vi "Attack.vi"(8 "error in (no error)":errorcluster, 9 "Attack?":T1, 10 "Team Index":i32, 11 "View":i32[](array[numeric])) -> (0 "error out":errorcluster, 1 "Direction":i32, 2 "Action":T2, 3 "View":i32[](array[numeric]), 4 "Enemy Found?":bool, 6 "Enemy Direction":i32)   [LabVIEW 2015, in "Common.lvlib"]
uses:
  Common.lvlib
  Type Defs/Action Enum.ctl
  Formics/Attack Options.ctl
  Type Defs/SB Type Defs.lvlib
  Formics/Formics.lvclass
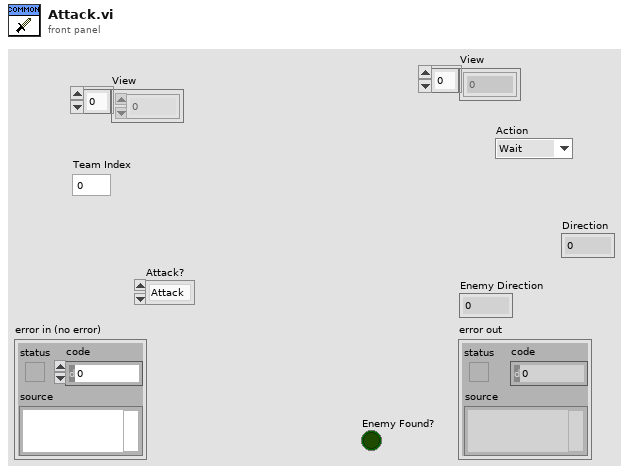
[diagram p1: front panel]
types:
  T1 = typedef "Formics.lvclass/Attack Options.ctl" = enum16{"Attack", "Run", "Distract"}
  T2 = typedef "SB Type Defs.lvlib/Action Enum.ctl" = enum16{"Wait", "Move", "Attack", "Replicate"}
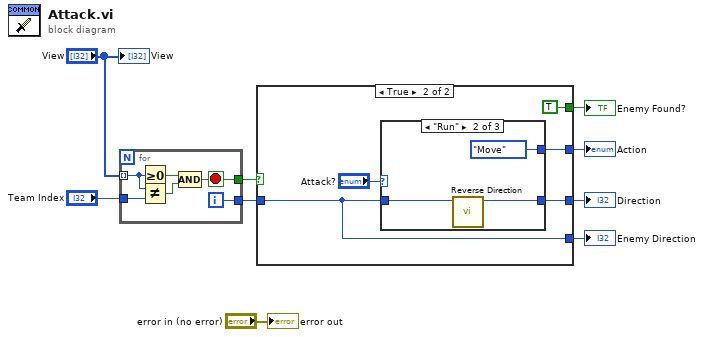
[diagram p0: block diagram]
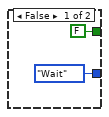
[diagram p2: hidden frame]
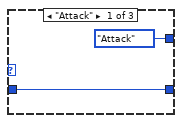
[diagram p3: hidden frame]
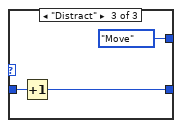
[diagram p4: hidden frame]
diagram:
  n1 = for {
    tunnel: "View" -> [w13] mode=indexing
    tunnel: "Team Index" -> [w14]
    tunnel: [w11] -> w2
    tunnel: [w10] -> w1
    i -> [w11]
    stop <- w10 stop-if-true
    n2 = Greater Or Equal To 0?(x=w13) -> (x >= 0?=w15:bool)
    n3 = Not Equal?(x=w13, y=w14) -> (x != y?=w12:bool)
    n4 = Compound Arithmetic op=AND(w15, w12) -> (w10:bool)
  }
  n5 = case shown="True" w1 {
    tunnel: [Action_Enum."Wait" ("Action") w22] -> w7
    tunnel: [_ w20] -> w8
    tunnel: [FALSE ("Enemy Found?") TRUE ("Enemy Found?")] -> w6
    tunnel: [_ w18] -> w5
    tunnel: w2 -> [_ w18]
    frame False {
    }
    frame True {
      n6 = case shown="\"Run\"" "Attack?" {
        tunnel: [Action_Enum."Attack" ("Action") Action_Enum."Move" ("Action") Action_Enum."Move" ("Action")] -> w22
        tunnel: [w23 w25 w28] -> w20
        tunnel: w18 -> [w23 w26 w29]
        frame "Attack" {
        }
        frame "Run" {
          n7 = call "Reverse Direction.vi"("Direction"=w26) -> ("Numeric"=w25:i32)  [unwired: 10 in]
        }
        frame "Distract" {
          n8 = Increment(x=w29) -> (x+1=w28:i32)
        }
      }
    }
  }
  "Action" <- w7
  "Direction" <- w8
  "Enemy Found?" <- w6
  "Enemy Direction" <- w5
  "error out" <- "error in (no error)"
  "View" <- "View"
